vi "Obtain Request Events.vi"(8 "error in":errorcluster, 10 "Create New? (F)":bool) -> (0 "error out":errorcluster, 2 "MainInterface Request Events":T1)   [LabVIEW 2018, in "MainInterface.lvlib"]
doc: "This VI Obtains/Creates the Requests events that will be used for other modules to communicate with the module that owns this VI. These Requests events will be accessed only via Public API methods for this module.\n\n<b>NOTE</b>: The contents of this VI are automatically generated and modified by the <b>Tools > DQMH Consortium > DQMH</b> utilities. Consider using those utilities instead of making your own modifications to this VI.\n_____\nBased on DQMH Project Template 7.0.1.1316."
uses:
  MainInterface.lvlib
  Request Events--cluster.ctl
  Stop Argument--cluster.ctl
  Show Panel Argument--cluster.ctl
  Hide Panel Argument--cluster.ctl
  Get Module Execution Status Argument--cluster.ctl
  Show Diagram Argument--cluster.ctl
  Register Window Argument--cluster.ctl
  <vilib>/Delacor/Delacor QMH/Libraries/Message Queue_class/Delacor_lib_QMH_Message Queue.lvclass
  Unregister Window Argument--cluster.ctl
  Is Window Opened Argument--cluster.ctl
  Is Window Opened (Reply Payload)--cluster.ctl
  Disbale Item Argument--cluster.ctl
  Enable Item Argument--cluster.ctl
panel:
  # "NOTE: The contents of this VI are automatically generated and modified by the Tools > DQMH Consortium > DQMH utilities. Consider using those utilities instead of making your own modifications to this VI."
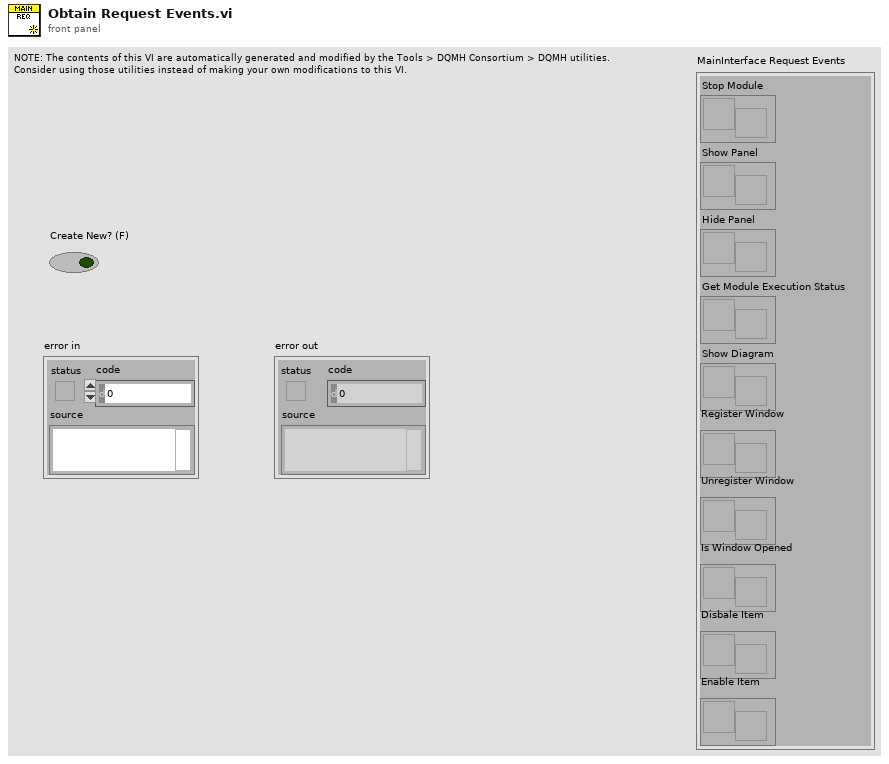
[diagram p1: front panel]
types:
  T1 = typedef "MainInterface.lvlib/Request Events--cluster.ctl" = cluster{"Stop Module":refnum<user-event>, "Show Panel":refnum<user-event>, "Hide Panel":refnum<user-event>, "Get Module Execution Status":refnum<user-event>, "Show Diagram":refnum<user-event>, "Register Window":refnum<user-event>, "Unregister Window":refnum<user-event>, "Is Window Opened":refnum<user-event>, "Disbale Item":refnum<user-event>, "Enable Item":refnum<user-event>}
  T2 = typedef "MainInterface.lvlib/Enable Item Argument--cluster.ctl" = cluster{"Module Name":string, "Item Name":string}
  T3 = typedef "MainInterface.lvlib/Disbale Item Argument--cluster.ctl" = cluster{"Module Name":string, "Item Name":string}
  T4 = typedef "MainInterface.lvlib/Is Window Opened Argument--cluster.ctl" = cluster{"Window Name":string, "Wait Notifier":refnum<notifier>, "wait for reply":bool}
  T5 = typedef "MainInterface.lvlib/Unregister Window Argument--cluster.ctl" = cluster{"Window Name":string}
  T6 = typedef "MainInterface.lvlib/Register Window Argument--cluster.ctl" = cluster{"Name":string, "Reference":refnum<vi>, "Message Queue":refnum<class "Delacor_lib_QMH_Message Queue.lvclass">}
  T7 = typedef "MainInterface.lvlib/Hide Panel Argument--cluster.ctl" = cluster{"Hide Panel?":bool}
  T8 = typedef "MainInterface.lvlib/Show Panel Argument--cluster.ctl" = cluster{"Show Panel?":bool}
  T9 = typedef "MainInterface.lvlib/Show Diagram Argument--cluster.ctl" = cluster{"Debug?":bool}
  T10 = typedef "MainInterface.lvlib/Get Module Execution Status Argument--cluster.ctl" = cluster{"Running?":bool}
  T11 = typedef "MainInterface.lvlib/Stop Argument--cluster.ctl" = cluster{"Origin":string, "Exit via Stop Module Req?":bool, "Wait for Module to stop?":bool}
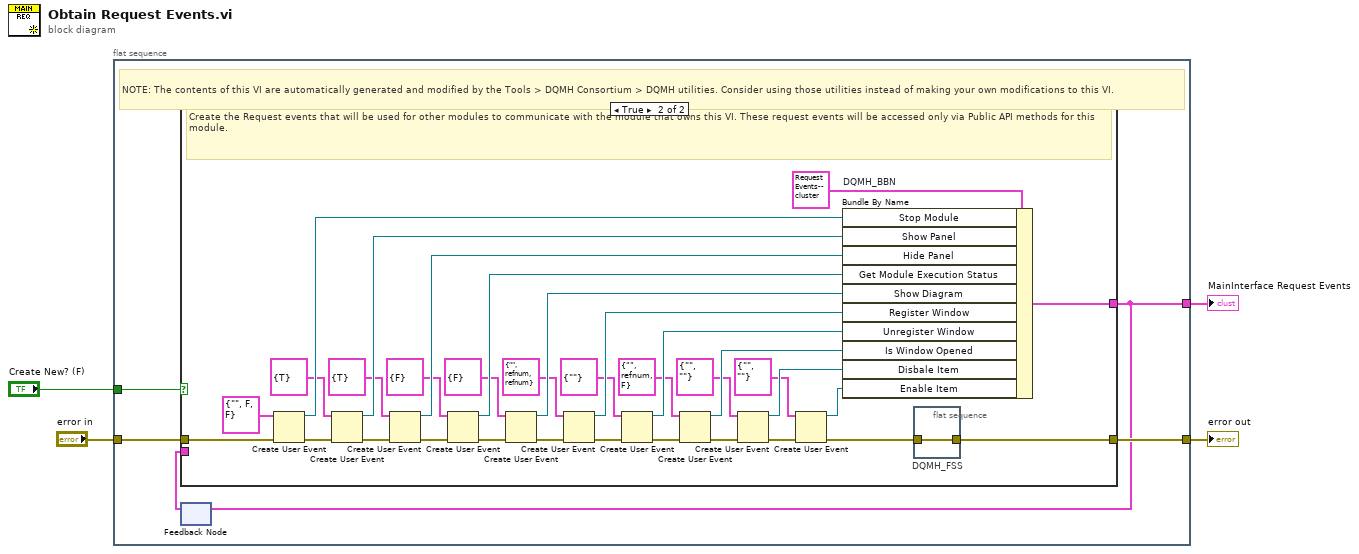
[diagram p0: block diagram]
diagram:
  n1 = flat-sequence {
    tunnel: [w9] -> w4
    tunnel: "error in" -> [w8]
    tunnel: [w6] -> w2
    tunnel: "Create New? (F)" -> [w5]
    frame #0 {
      # "NOTE: The contents of this VI are automatically generated and modified by the Tools > DQMH Consortium > DQMH utilities. Consider using those utilities instead of making your own modifications to this VI."
      n2 = feedback #1() -> (w7:T1)  [unwired: 1 in]
      n3 = case shown="True" w5 {
        tunnel: [w10 w35] -> w9
        tunnel: w8 -> [w10 w45]
        tunnel: [w11 w42] -> w6
        tunnel: w7 -> [w11 _]
        frame False {
          # "Obtain the Request events that were created in a previous call to this VI."
        }
        frame True {
          # "Create the Request events that will be used for other modules to communicate with the module that owns this VI. These request events will be accessed only via Public API methods for this module."
          n4 = Create User Event(user event datatype=T11 {"Origin"="", "Exit via Stop Module Req?"=FALSE, "Wait for Module to stop?"=FALSE} ("Stop Argument"), error in=w45) -> (user event=w43:refnum<user-event>, error out=w40:errorcluster)
          n5 = Create User Event(user event datatype=T8 {"Show Panel?"=TRUE} ("Show Panel Argument"), error in=w40) -> (user event=w39:refnum<user-event>, error out=w38:errorcluster)
          n6 = Create User Event(user event datatype=T7 {"Hide Panel?"=TRUE} ("Hide Panel Argument"), error in=w38) -> (user event=w37:refnum<user-event>, error out=w36:errorcluster)
          n7 = Create User Event(user event datatype=T10 {"Running?"=FALSE} ("Get Module Execution Status Argument"), error in=w36) -> (user event=w33:refnum<user-event>, error out=w34:errorcluster)
          n8 = Create User Event(user event datatype=T9 {"Debug?"=FALSE} ("Show Diagram Argument"), error in=w34) -> (user event=w30:refnum<user-event>, error out=w31:errorcluster)
          n9 = Create User Event(user event datatype=T6 {"Name"="", "Reference"=refnum, "Message Queue"=refnum} ("Register Window Argument"), error in=w31) -> (user event=w25:refnum<user-event>, error out=w26:errorcluster)
          n10 = Create User Event(user event datatype=T5 {"Window Name"=""} ("Unregister Window Argument"), error in=w26) -> (user event=w22:refnum<user-event>, error out=w23:errorcluster)
          n11 = Create User Event(user event datatype=T4 {"Window Name"="", "Wait Notifier"=refnum, "wait for reply"=FALSE} ("Is Window Opened Argument"), error in=w23) -> (user event=w19:refnum<user-event>, error out=w20:errorcluster)
          n12 = Create User Event(user event datatype=T3 {"Module Name"="", "Item Name"=""} ("Disbale Item Argument"), error in=w20) -> (user event=w16:refnum<user-event>, error out=w17:errorcluster)
          n13 = Create User Event(user event datatype=T2 {"Module Name"="", "Item Name"=""} ("Enable Item Argument"), error in=w17) -> (user event=w13:refnum<user-event>, error out=w14:errorcluster)
          n14 = Bundle By Name "DQMH_BBN"(cluster=T1 {"Stop Module"=refnum, "Show Panel"=refnum, "Hide Panel"=refnum, "Get Module Execution Status"=refnum, "Show Diagram"=refnum, "Register Window"=refnum, "Unregister Window"=refnum, "Is Window Opened"=refnum, "Disbale Item"=refnum, "Enable Item"=refnum} ("output cluster"), "Stop Module"=w43, "Show Panel"=w39, "Hide Panel"=w37, "Get Module Execution Status"=w33, "Show Diagram"=w30, "Register Window"=w25, "Unregister Window"=w22, "Is Window Opened"=w19, "Disbale Item"=w16, "Enable Item"=w13) -> (w42:T1)
          n15 = flat-sequence "DQMH_FSS" {
            tunnel: w14 -> [w46]
            tunnel: [w46] -> w35
            frame #0 {
            }
          }
        }
      }
      n16 = feedback-in #1(w6) -> ()
    }
  }
  "MainInterface Request Events" <- w2
  "error out" <- w4
